vi "Check Limit.vi"(8 "error in (no error)":errorcluster, 9 "Distance (mm)":dbl, 10 "Axis":T1=enum."Y", 11 "Stage Controller in":refnum<class "Stage Controller.lvclass">) -> (0 "error out":errorcluster, 3 "Stage Controller out":refnum<class "Stage Controller.lvclass">)   [LabVIEW 2018, in "Stage Controller.lvlib" / "Stage Controller.lvclass"]
uses:
  Stage Controller.lvclass
  Stage Axis.ctl
  Stage Controller.lvclass/Stage Controller.ctl
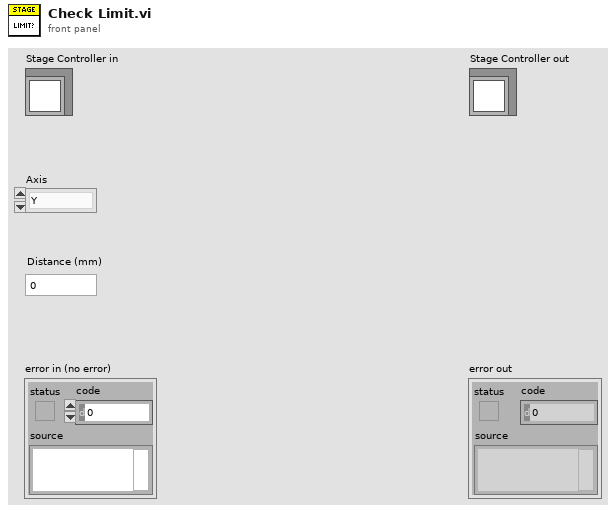
[diagram p1: front panel]
types:
  T1 = typedef "Stage Controller.lvlib/Stage Controller.lvclass/Stage Axis.ctl" = enum16{"unspecified", "X", "Y", "Z"}
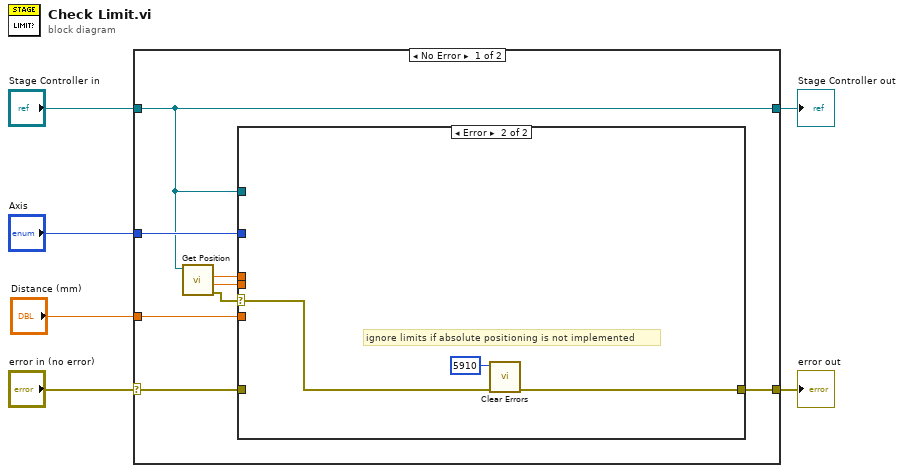
[diagram p0: block diagram]
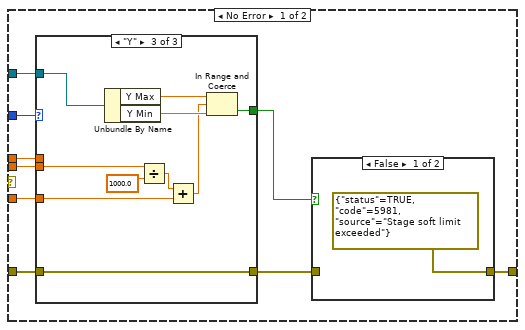
[diagram p2: hidden frame]
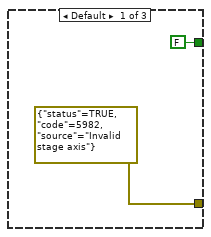
[diagram p3: hidden frame]
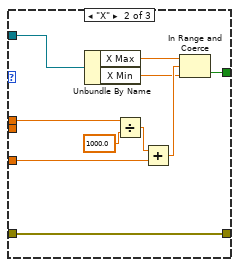
[diagram p4: hidden frame]
diagram:
  n1 = case shown="No Error" "error in (no error)" {
    selector: "error in (no error)" -> [w10 w52]
    tunnel: [w14 w52] -> w5
    tunnel: [w12 w51] -> w3
    tunnel: "Stage Controller in" -> [w12 w51]
    tunnel: "Distance (mm)" -> [w11 _]
    tunnel: "Axis" -> [w13 _]
    frame No Error {
      n2 = call-dynamic "Get Position.vi"("Stage Controller in"=w12) -> ("error out"=w7:errorcluster, "Y (mm)"=w9:dbl, "X (mm)"=w8:dbl)  [unwired: 6 in, 2 out]
      n3 = case shown="Error" w7 {
        selector: w7 -> [_ w50]
        tunnel: [w23 w49] -> w14
        tunnel: w13 -> [w22 _]
        tunnel: w12 -> [w21 _]
        tunnel: w11 -> [w20 _]
        tunnel: w10 -> [w18 _]
        tunnel: w9 -> [w16 _]
        tunnel: w8 -> [w15 _]
        frame No Error {
          n4 = case shown="\"Y\"" w22 {
            tunnel: w21 -> [_ w31 w45]
            tunnel: w20 -> [_ w32 w44]
            tunnel: [FALSE w30 w40] -> w19
            tunnel: w18 -> [_ w29 w39]
            tunnel: [errorcluster {"status"=TRUE, "code"=5982, "source"="Invalid stage axis"} ("error constant") w29 w39] -> w17
            tunnel: w16 -> [_ _ w36]
            tunnel: w15 -> [_ w26 _]
            frame Default {
            }
            frame "X" {
              n5 = Unbundle By Name(w31) -> ("X Max"=w33:dbl, "X Min"=w34:dbl)
              n6 = Divide(x=w26, y=1000.0) -> (x/y=w28:dbl)
              n7 = Add(x=w28, y=w32) -> (x+y=w35:dbl)
              n8 = In Range and Coerce(upper limit=w33, x=w35, lower limit=w34) -> (In Range?=w30:bool)  [unwired: 1 out]
            }
            frame "Y" {
              n9 = Unbundle By Name(w45) -> ("Y Max"=w43:dbl, "Y Min"=w42:dbl)
              n10 = Divide(x=w36, y=1000.0) -> (x/y=w38:dbl)
              n11 = Add(x=w38, y=w44) -> (x+y=w41:dbl)
              n12 = In Range and Coerce(upper limit=w43, x=w41, lower limit=w42) -> (In Range?=w40:bool)  [unwired: 1 out]
            }
          }
          n13 = case shown="False" w19 {
            tunnel: w17 -> [_ w47]
            tunnel: [errorcluster {"status"=TRUE, "code"=5981, "source"="Stage soft limit exceeded"} ("error constant") w47] -> w23
            frame False {
            }
            frame True {
            }
          }
        }
        frame Error {
          # "ignore limits if absolute positioning is not implemented"
          n14 = call <vilib>:"Clear Errors.vi"("error in (no error)"=w50, "specific error code to clear (0: all)"=5910) -> ("error out"=w49:errorcluster)  [unwired: 4 in, 1 out]
        }
      }
    }
    frame Error {
    }
  }
  "error out" <- w5
  "Stage Controller out" <- w3
